vi "Monitor.vi"() -> ()   [LabVIEW 2017]
uses:
  Control_Figura.ctl
  Control_Eje_Figura.ctl
  Control_Operacion.ctl
  Control_Selector_Variable.ctl
  Control_Opciones.ctl
  <vilib>/Motion/Express/_s/nimc.fb.read.readExecutionData.axis.vi
  <vilib>/Motion/BlockNode/FB.NIMotion.xnode
panel:
  out "3D Picture":refnum<vi>(3d-picture)
  in  "Objetos":path=path "C:/Users/LuisFernando/Documents/UPIITA/8vo semestre/Instrumentacion Virtual Aplicada/Solidworks/2_Ejes_Figuras/Figuras"
  in  "Mundo":path=path "C:/Users/LuisFernando/Documents/UPIITA/8vo semestre/Instrumentacion Virtual Aplicada/Solidworks/2_Ejes_Figuras/Mundo.wrl"
  in  "Selector de Variable":T1=enum."Velocidades"
  in  "Tab Control":enum32{"Eje X", "Eje Y", "Eje Z"}(tab)
  out "Valor X":dbl=3.0
  out "Velocidad X":dbl=3.0
  out "Posición X":dbl=1284.670631579
  out "Velocidad X":dbl(graph)=3.0
  out "Posición X":dbl(graph)=1284.670631579
  in  "Actualizar_Eje_X":bool
  in  "Figura Geometrica X":T2
  in  "Eje de la Figura X":T3
  in  "Operación X":T4=enum."Translación"
  out "Valor Y":dbl=8.0
  out "Velocidad Y":dbl=8.0
  out "Posición Y":dbl=1275.193684211
  out "Velocidad Y":dbl(graph)=8.0
  out "Posición Y":dbl(graph)=1275.193684211
  in  "Actualizar_Eje_Y":bool
  in  "Figura Geometrica Y":T2
  in  "Eje de la Figura Y":T3=enum."Y"
  in  "Operación Y":T4=enum."Translación"
  out "Valor Z":dbl=1.0
  out "Velocidad Z":dbl=1.0
  out "Posición Z":dbl=787.306635341
  out "Velocidad Z":dbl(graph)=1.0
  out "Posición Z":dbl(graph)=787.306635341
  in  "Actualizar_Eje_Z":bool
  in  "Figura Geometrica Z":T2
  in  "Eje de la Figura Z":T3=enum."Z"
  in  "Operación Z":T4=enum."Translación"
  in  "Stop Button":bool
  in  "Panel de Monitoreo":enum32{"Posición", "Velocidad"}(tab)=enum."Velocidad"
  out "Posición 3":dbl(graph)=787.306635341
  out "Posición 2":dbl(graph)=1275.193684211
  out "Posición 1":dbl(graph)=1284.670631579
  out "Velocidad 3":dbl(graph)=1.0
  out "Velocidad 2":dbl(graph)=8.0
  out "Velocidad 1":dbl(graph)=3.0
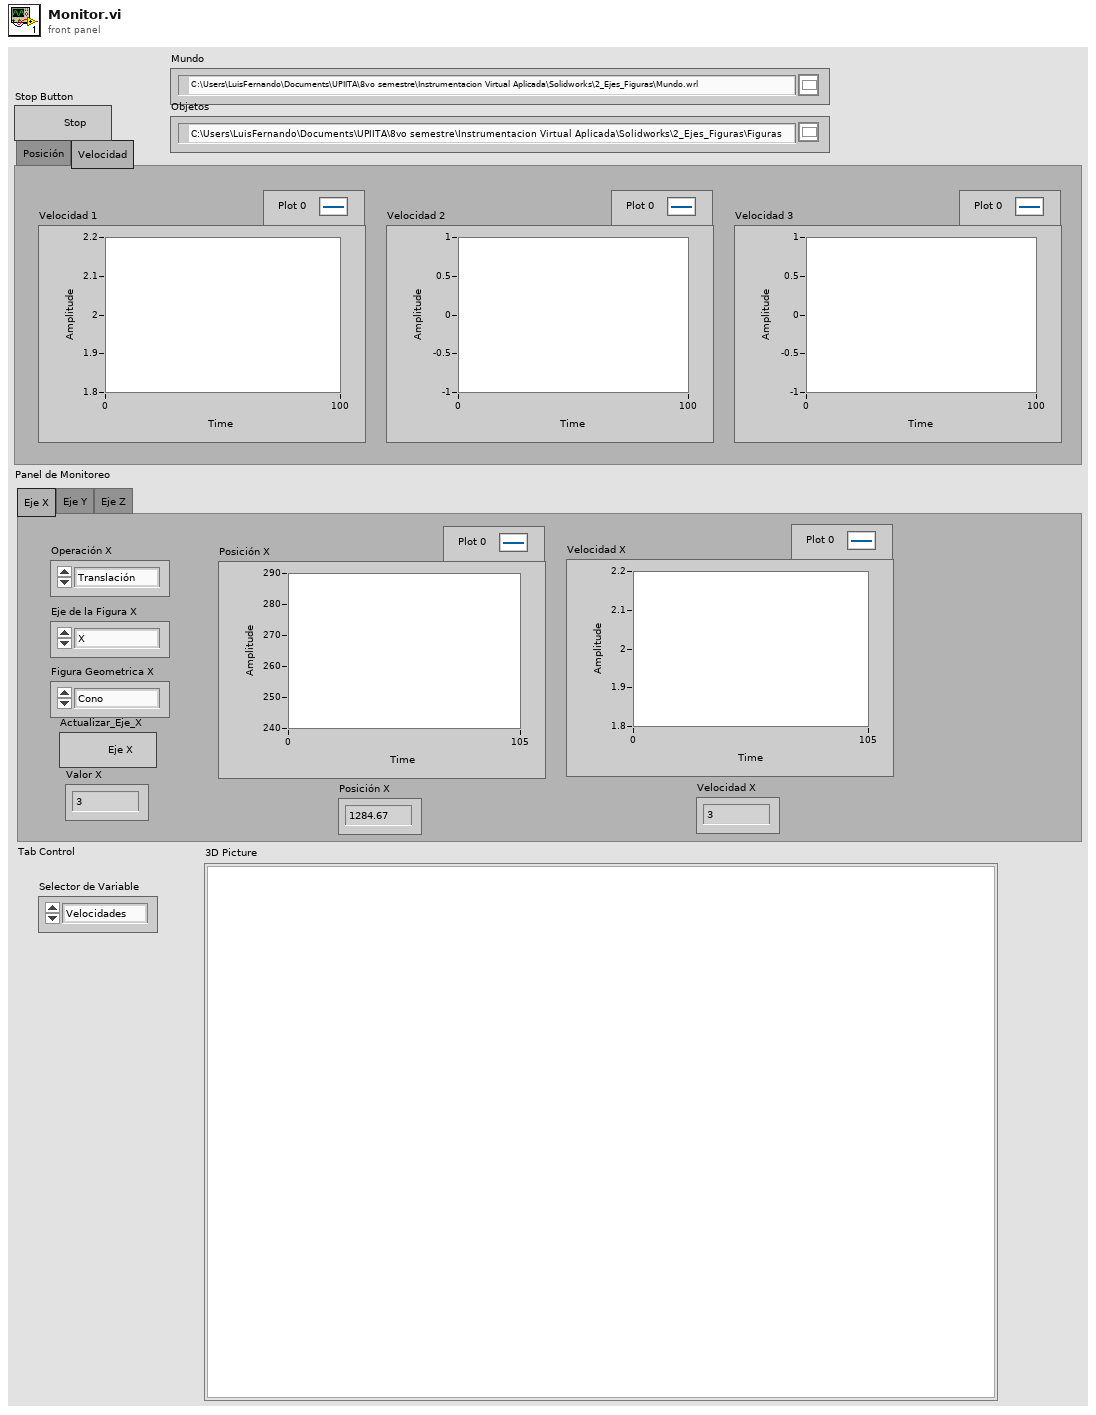
[diagram p1: front panel]
types:
  T1 = typedef "Control_Selector_Variable.ctl" = enum16{"Posiciones", "Velocidades"}
  T2 = typedef "Control_Figura.ctl" = enum16{"Cono", "Esfera", "Cilindro"}
  T3 = typedef "Control_Eje_Figura.ctl" = enum16{"X", "Y", "Z"}
  T4 = typedef "Control_Operacion.ctl" = enum16{"Escala", "Translación", "Rotación"}
  T5 = typedef "Control_Opciones.ctl" = cluster{"Opción X":i32, "Opción Y":i32, "Opción Z":i32, "Posición X":dbl, "Velocidad X":dbl, "Posición Y":dbl, "Velocidad Y":dbl, "Posición Z":dbl, "Velocidad Z":dbl, "Escala":dbl[][], "Translación":dbl[][], "Rotación":dbl[][], "Operacion SX":T4, "Eje de la Figura SX":T3, "Figura Geométrica SX":T2, "Operacion SY":T4, "Eje de la Figura SY":T3, "Figura Geométrica SY":T2, "Operacion SZ":T4, "Eje de la Figura SZ":T3, "Figura Geométrica SZ":T2}
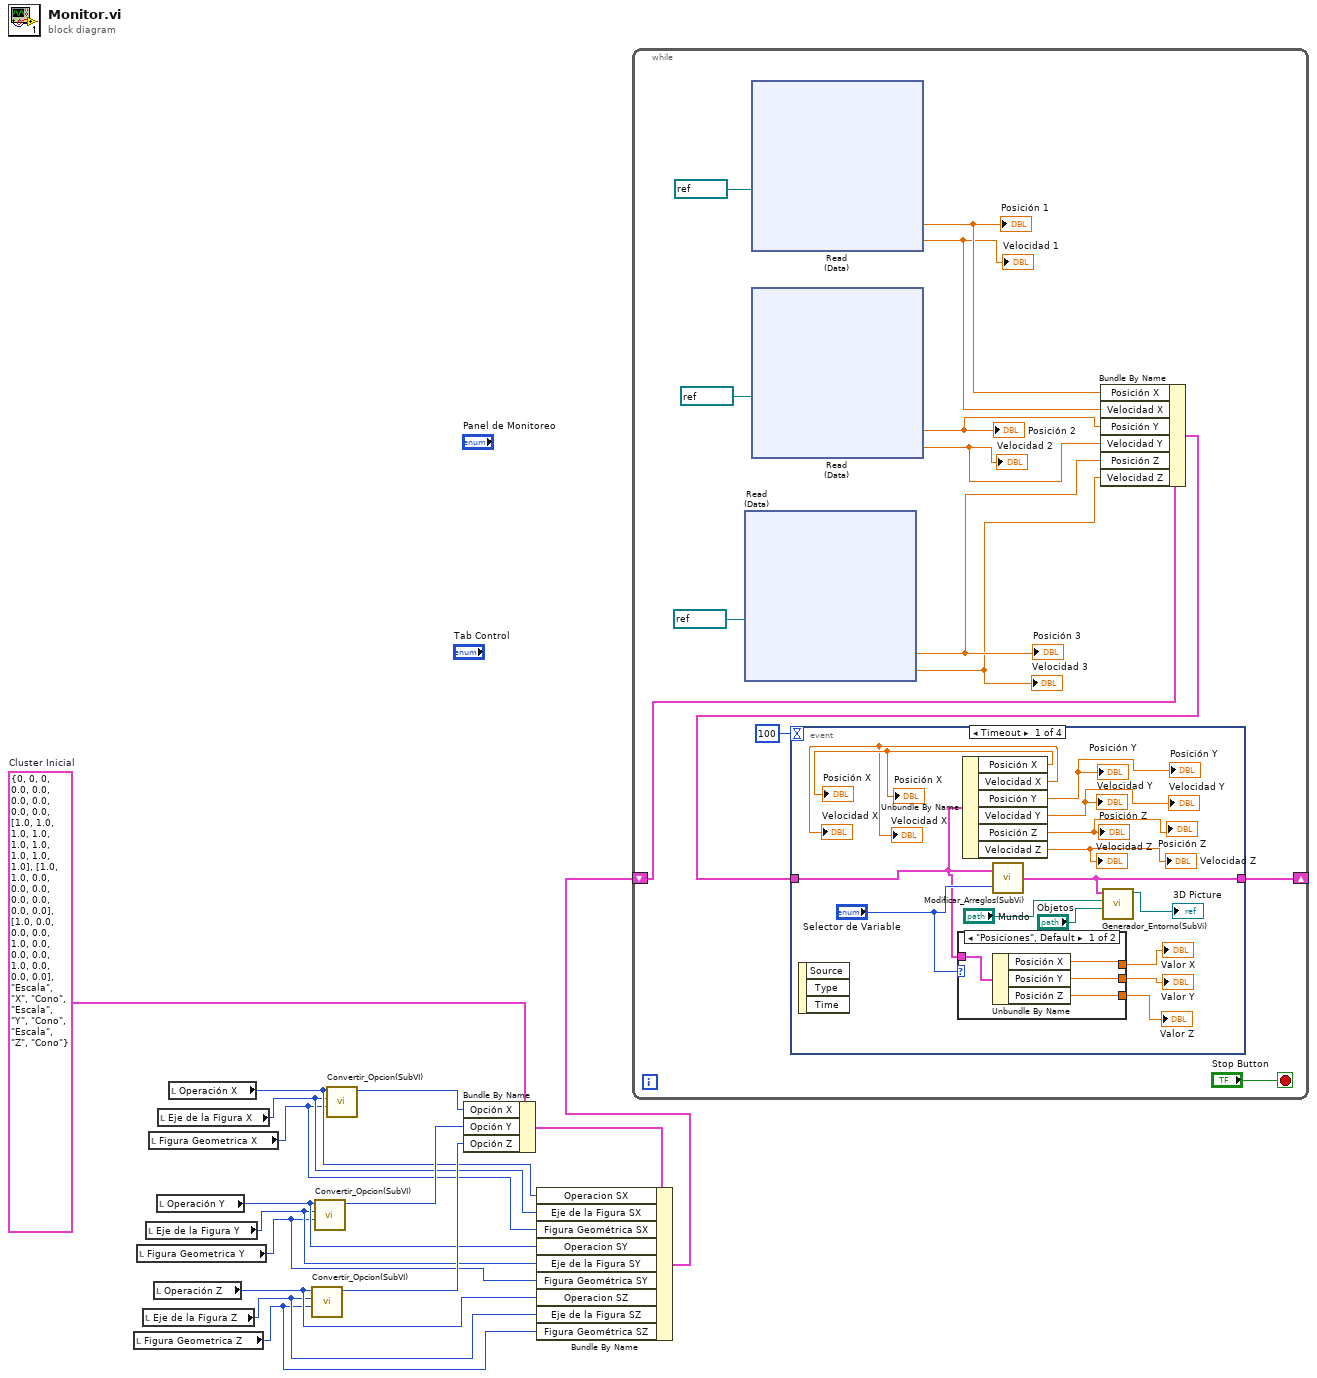
[diagram p0: block diagram]
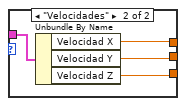
[diagram p2: hidden frame]
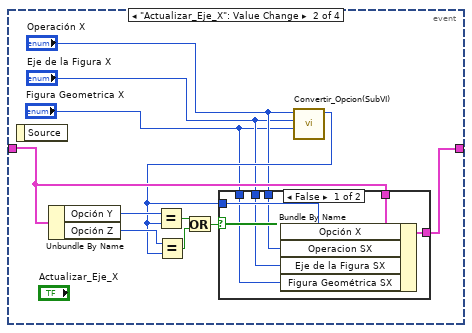
[diagram p3: hidden frame]
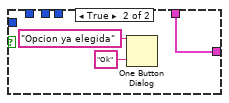
[diagram p4: hidden frame]
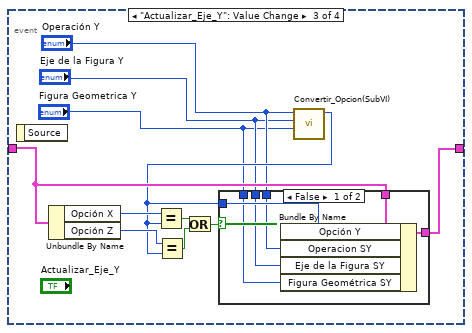
[diagram p5: hidden frame]
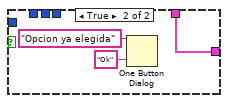
[diagram p6: hidden frame]
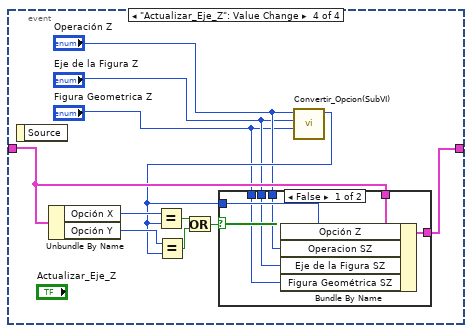
[diagram p7: hidden frame]
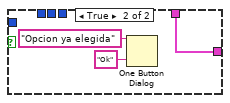
[diagram p8: hidden frame]
diagram:
  w15 = T5 {"Opción X"=0, "Opción Y"=0, "Opción Z"=0, "Posición X"=0.0, "Velocidad X"=0.0, "Posición Y"=0.0, "Velocidad Y"=0.0, "Posición Z"=0.0, "Velocidad Z"=0.0, "Escala"=[[1.0, 1.0, 1.0], [1.0, 1.0, 1.0], [1.0, 1.0, 1.0]], "Translación"=[[1.0, 1.0, 0.0], [0.0, 0.0, 0.0], [0.0, 0.0, 0.0]], "Rotación"=[[1.0, 0.0, 0.0, 0.0], [1.0, 0.0, 0.0, 0.0], [1.0, 0.0, 0.0, 0.0]], "Operacion SX"=enum."Escala", "Eje de la Figura SX"=enum."X", "Figura Geométrica SX"=enum."Cono", "Operacion SY"=enum."Escala", "Eje de la Figura SY"=enum."Y", "Figura Geométrica SY"=enum."Cono", "Operacion SZ"=enum."Escala", "Eje de la Figura SZ"=enum."Z", "Figura Geométrica SZ"=enum."Cono"}  # Cluster Inicial
  n1 = local read "Figura Geometrica Z"() -> (w1:T2)
  n2 = local read "Figura Geometrica Y"() -> (w4:T2)
  n3 = local read "Eje de la Figura Z"() -> (w2:T3)
  n4 = local read "Eje de la Figura Y"() -> (w5:T3)
  n5 = local read "Figura Geometrica X"() -> (w7:T2)
  n6 = local read "Operación Z"() -> (w3:T4)
  n7 = local read "Operación Y"() -> (w6:T4)
  n8 = local read "Eje de la Figura X"() -> (w8:T3)
  n9 = local read "Operación X"() -> (w9:T4)
  n10 = call "Convertir_Opcion(SubVI).vi"("Figura Geometrica X"=w1, "Eje de la Figura X"=w2, "Operación X"=w3) -> ("Numeric Control"=w12:i32)  [unwired: 8 in]
  n11 = call "Convertir_Opcion(SubVI).vi"("Figura Geometrica X"=w4, "Eje de la Figura X"=w5, "Operación X"=w6) -> ("Numeric Control"=w13:i32)  [unwired: 8 in]
  n12 = call "Convertir_Opcion(SubVI).vi"("Figura Geometrica X"=w7, "Eje de la Figura X"=w8, "Operación X"=w9) -> ("Numeric Control"=w14:i32)  [unwired: 8 in]
  n13 = Bundle By Name(cluster=w15, "Opción X"=w14, "Opción Y"=w13, "Opción Z"=w12) -> (w11:T5)
  n14 = Bundle By Name(cluster=w11, "Operacion SX"=w9, "Eje de la Figura SX"=w8, "Figura Geométrica SX"=w7, "Operacion SY"=w6, "Eje de la Figura SY"=w5, "Figura Geométrica SY"=w4, "Operacion SZ"=w3, "Eje de la Figura SZ"=w2, "Figura Geométrica SZ"=w1) -> (w10:T5)
  n15 = while {
    shift-right: [w25] -> _
    shift-left: w10 -> [w17]
    stop <- "Stop Button" stop-if-true
    n16 = xnode "Read\n(Data)"("resource"=refnum<k21> "Eje Z") -> ("position"=w19:dbl, "velocity"=w18:dbl)  [unwired: 1 in, 3 out]
    "Posición 3" <- w19
    "Velocidad 3" <- w18
    n17 = xnode "Read\n(Data)"("resource"=refnum<k21> "EJE X") -> ("position"=w23:dbl, "velocity"=w22:dbl)  [unwired: 1 in, 3 out]
    "Posición 1" <- w23
    "Velocidad 1" <- w22
    n18 = xnode "Read\n(Data)"("resource"=refnum<k21> "EJE Y") -> ("position"=w21:dbl, "velocity"=w20:dbl)  [unwired: 1 in, 3 out]
    "Posición 2" <- w21
    "Velocidad 2" <- w20
    n19 = Bundle By Name(cluster=w17, "Posición X"=w23, "Velocidad X"=w22, "Posición Y"=w21, "Velocidad Y"=w20, "Posición Z"=w19, "Velocidad Z"=w18) -> (w16:T5)
    n20 = event shown="[0] Timeout" {
      selector: _ -> [_ _ _ _]
      dyn-events: _ -> [_ _ _ _]
      timeout: 100 -> [_ _ _ _]
      tunnel: w16 -> [w40 w57 w77 w97]
      tunnel: [w33 w58 w78 w98] -> w25
      event Timeout {
        n21 = event-data() -> ()  [unwired: 1 in, 3 out]
        n22 = case shown="\"Posiciones\", Default" "Selector de Variable" {
          tunnel: w40 -> [w48 w52]
          tunnel: [w47 w51] -> w41
          tunnel: [w46 w50] -> w42
          tunnel: [w45 w49] -> w43
          frame "Posiciones", Default {
            n23 = Unbundle By Name(w48) -> ("Posición X"=w47:dbl, "Posición Y"=w46:dbl, "Posición Z"=w45:dbl)
          }
          frame "Velocidades" {
            n24 = Unbundle By Name(w52) -> ("Velocidad X"=w51:dbl, "Velocidad Y"=w50:dbl, "Velocidad Z"=w49:dbl)
          }
        }
        "Valor Z" <- w43
        "Valor Y" <- w42
        "Valor X" <- w41
        n25 = Unbundle By Name(w40) -> ("Posición X"=→"Posición X" →"Posición X":dbl, "Velocidad X"=→"Velocidad X" →"Velocidad X":dbl, "Posición Y"=→"Posición Y" →"Posición Y":dbl, "Velocidad Y"=→"Velocidad Y" →"Velocidad Y":dbl, "Posición Z"=→"Posición Z" →"Posición Z":dbl, "Velocidad Z"=→"Velocidad Z" →"Velocidad Z":dbl)
        n26 = call "Modificar_Arreglos(SubVi).vi"("Selector de Variable"="Selector de Variable", "input cluster"=w40) -> ("output cluster"=w33:T5)
        n27 = call "Generador_Entorno(SubVi).vi"("Objetos"="Objetos", "Mundo"="Mundo", "Cluster"=w33) -> ("3D Picture"=→"3D Picture":refnum<vi>)  [unwired: 8 in]
      }
      event "Actualizar_Eje_X": Value Change {
        n28 = event-data() -> ()  [unwired: 1 in, 1 out]
        n29 = Unbundle By Name(w57) -> ("Opción Y"=w63:i32, "Opción Z"=w62:i32)
        n30 = call "Convertir_Opcion(SubVI).vi"("Figura Geometrica X"="Figura Geometrica X", "Eje de la Figura X"="Eje de la Figura X", "Operación X"="Operación X") -> ("Numeric Control"=w56:i32)  [unwired: 8 in]
        n31 = Equal?(x=w63, y=w56) -> (x = y?=w61:bool)
        n32 = Equal?(x=w62, y=w56) -> (x = y?=w60:bool)
        n33 = Or(x=w61, y=w60) -> (x .or. y?=w59:bool)
        n34 = case shown="False" w59 {
          tunnel: [w69 w72] -> w58
          tunnel: w57 -> [w68 w72]
          tunnel: w56 -> [w67 _]
          tunnel: "Operación X" -> [w66 _]
          tunnel: "Eje de la Figura X" -> [w65 _]
          tunnel: "Figura Geometrica X" -> [w64 _]
          frame False {
            n35 = Bundle By Name(cluster=w68, "Opción X"=w67, "Operacion SX"=w66, "Eje de la Figura SX"=w65, "Figura Geométrica SX"=w64) -> (w69:T5)
          }
          frame True {
            n36 = One Button Dialog(message="Opcion ya elegida", button name ("OK")="Ok") -> ()  [unwired: 1 out]
          }
        }
      }
      event "Actualizar_Eje_Y": Value Change {
        n37 = event-data() -> ()  [unwired: 1 in, 1 out]
        n38 = Unbundle By Name(w77) -> ("Opción X"=w83:i32, "Opción Z"=w82:i32)
        n39 = call "Convertir_Opcion(SubVI).vi"("Figura Geometrica X"="Figura Geometrica Y", "Eje de la Figura X"="Eje de la Figura Y", "Operación X"="Operación Y") -> ("Numeric Control"=w76:i32)  [unwired: 8 in]
        n40 = Equal?(x=w83, y=w76) -> (x = y?=w81:bool)
        n41 = Equal?(x=w82, y=w76) -> (x = y?=w80:bool)
        n42 = Or(x=w81, y=w80) -> (x .or. y?=w79:bool)
        n43 = case shown="False" w79 {
          tunnel: [w89 w92] -> w78
          tunnel: w77 -> [w88 w92]
          tunnel: w76 -> [w87 _]
          tunnel: "Operación Y" -> [w86 _]
          tunnel: "Eje de la Figura Y" -> [w85 _]
          tunnel: "Figura Geometrica Y" -> [w84 _]
          frame False {
            n44 = Bundle By Name(cluster=w88, "Opción Y"=w87, "Operacion SY"=w86, "Eje de la Figura SY"=w85, "Figura Geométrica SY"=w84) -> (w89:T5)
          }
          frame True {
            n45 = One Button Dialog(message="Opcion ya elegida", button name ("OK")="Ok") -> ()  [unwired: 1 out]
          }
        }
      }
      event "Actualizar_Eje_Z": Value Change {
        n46 = event-data() -> ()  [unwired: 1 in, 1 out]
        n47 = Unbundle By Name(w97) -> ("Opción X"=w103:i32, "Opción Y"=w102:i32)
        n48 = call "Convertir_Opcion(SubVI).vi"("Figura Geometrica X"="Figura Geometrica Z", "Eje de la Figura X"="Eje de la Figura Z", "Operación X"="Operación Z") -> ("Numeric Control"=w96:i32)  [unwired: 8 in]
        n49 = Equal?(x=w103, y=w96) -> (x = y?=w101:bool)
        n50 = Equal?(x=w102, y=w96) -> (x = y?=w100:bool)
        n51 = Or(x=w101, y=w100) -> (x .or. y?=w99:bool)
        n52 = case shown="False" w99 {
          tunnel: [w109 w112] -> w98
          tunnel: w97 -> [w108 w112]
          tunnel: w96 -> [w107 _]
          tunnel: "Operación Z" -> [w106 _]
          tunnel: "Eje de la Figura Z" -> [w105 _]
          tunnel: "Figura Geometrica Z" -> [w104 _]
          frame False {
            n53 = Bundle By Name(cluster=w108, "Opción Z"=w107, "Operacion SZ"=w106, "Eje de la Figura SZ"=w105, "Figura Geométrica SZ"=w104) -> (w109:T5)
          }
          frame True {
            n54 = One Button Dialog(message="Opcion ya elegida", button name ("OK")="Ok") -> ()  [unwired: 1 out]
          }
        }
      }
    }
  }
